vi "Analysis Configuration Dialog.vi"(11 "Data In":T1={"UI References"={"Exit Ref"=refnum, "Save Ref"=refnum, "Open Ref"=refnum, "Export Ref"=refnum, "Acquire Ref"=refnum, "Configure Ref"=refnum, "Graph Ref"=refnum, "Clear Ref"=refnum, "Analyze Ref"=refnum, "Status Ref"=refnum, "Snapshot Ref"=refnum}, "User Specified"={"Hardware Configuration"={"Signal Channel"="PXI1Slot7/ao0", "Response Channel"="PXI1Slot7/ai0", "Trigger Channel"="/PXI1Slot7/PFI0", "Number of Acquisitions"=1.0}, "Analysis Configuration"={"Statistics"=TRUE}, "Signal Type"=enum."From Excel", "New Data Behavior"=enum."Replace", "Signal Configuration"={"Chirp Amplitude"=0.0, "I/O Limit"=0.0, "Sample Rate"=0.0, "Chirp Duration (s)"=0.0, "Upper Frequency"=0.0, "Lower Frequency"=0.0, "Windowing"=enum."None"}, "Waveform File"="", "Save Location"=""}}) -> (3 "Data Out":T1={"UI References"={"Exit Ref"=refnum, "Save Ref"=refnum, "Open Ref"=refnum, "Export Ref"=refnum, "Acquire Ref"=refnum, "Configure Ref"=refnum, "Graph Ref"=refnum, "Clear Ref"=refnum, "Analyze Ref"=refnum, "Status Ref"=refnum, "Snapshot Ref"=refnum}, "User Specified"={"Hardware Configuration"={"Signal Channel"="PXI1Slot7/ao0", "Response Channel"="PXI1Slot7/ai0", "Trigger Channel"="/PXI1Slot7/PFI0", "Number of Acquisitions"=1.0}, "Analysis Configuration"={"Statistics"=TRUE}, "Signal Type"=enum."From Excel", "New Data Behavior"=enum."Replace", "Signal Configuration"={"Chirp Amplitude"=0.0, "I/O Limit"=0.0, "Sample Rate"=0.0, "Chirp Duration (s)"=0.0, "Upper Frequency"=0.0, "Lower Frequency"=0.0, "Windowing"=enum."None"}, "Waveform File"="", "Save Location"=""}})   [LabVIEW 2017]
doc: "Displays the analysis configuration dialog if the user has the \"Prompt?\" preference set."
uses:
  controls/Data.ctl
  controls/UI References.ctl
  controls/HW Configuration.ctl
  controls/Analysis Configuration.ctl
  controls/New Data Behavior.ctl
  controls/Signal Configuration.ctl
panel:
  # "(Scroll up to see large state data in/out clusters)"
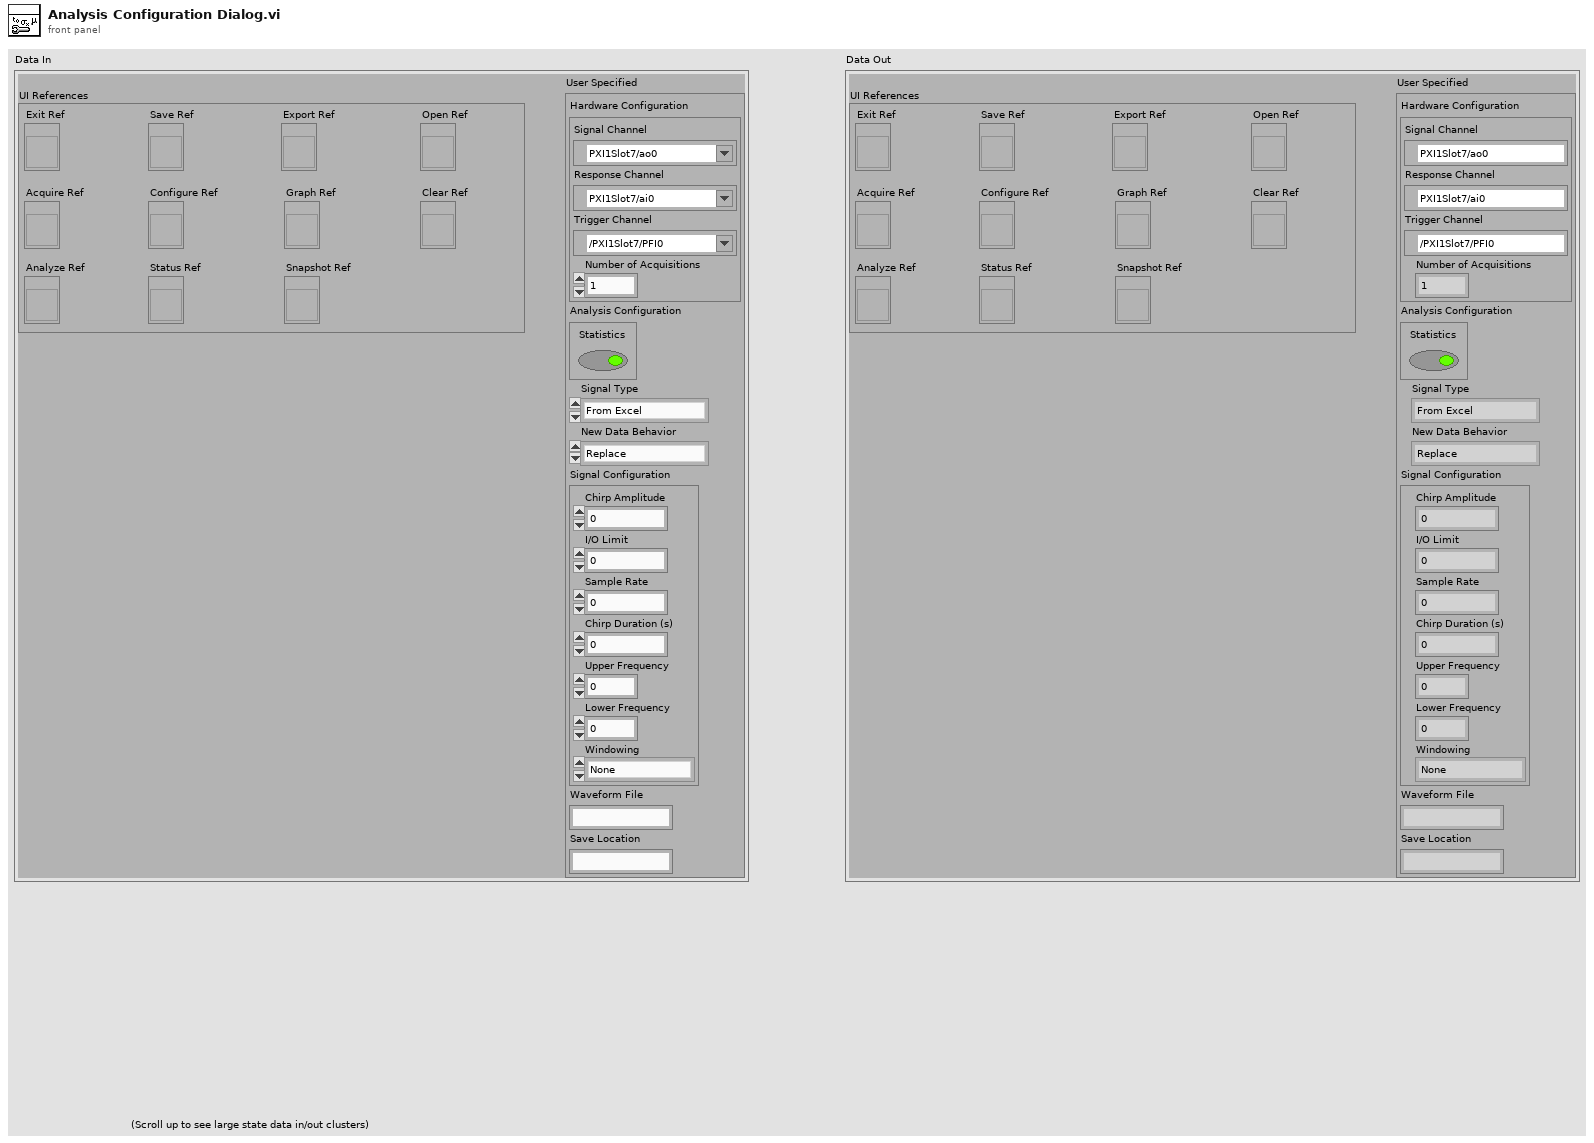
[diagram p1: front panel]
types:
  T1 = typedef "Data.ctl" = cluster{"UI References":T2, "User Specified":cluster{"Hardware Configuration":T3, "Analysis Configuration":T4, "Signal Type":enum16{"From Excel", "Single Chirp"}, "New Data Behavior":T5, "Signal Configuration":T6, "Waveform File":string, "Save Location":string}}
  T2 = typedef "UI References.ctl" = cluster{"Exit Ref":refnum<vi>, "Save Ref":refnum<vi>, "Open Ref":refnum<vi>, "Export Ref":refnum<vi>, "Acquire Ref":refnum<vi>, "Configure Ref":refnum<vi>, "Graph Ref":refnum<vi>, "Clear Ref":refnum<vi>, "Analyze Ref":refnum<vi>, "Status Ref":refnum<vi>, "Snapshot Ref":refnum<vi>}
  T3 = typedef "HW Configuration.ctl" = cluster{"Signal Channel":tag, "Response Channel":tag, "Trigger Channel":tag, "Number of Acquisitions":dbl}
  T4 = typedef "Analysis Configuration.ctl" = cluster{"Statistics":bool}
  T5 = typedef "New Data Behavior.ctl" = enum16{"Replace", "Overlay", "Append"}
  T6 = typedef "Signal Configuration.ctl" = cluster{"Chirp Amplitude":dbl, "I/O Limit":dbl, "Sample Rate":dbl, "Chirp Duration (s)":dbl, "Upper Frequency":dbl, "Lower Frequency":dbl, "Windowing":enum16{"None", "Exponential", "Flat top", "Hamming", "Hanning", "Kaiser-Bessel", "Rectangular"}}
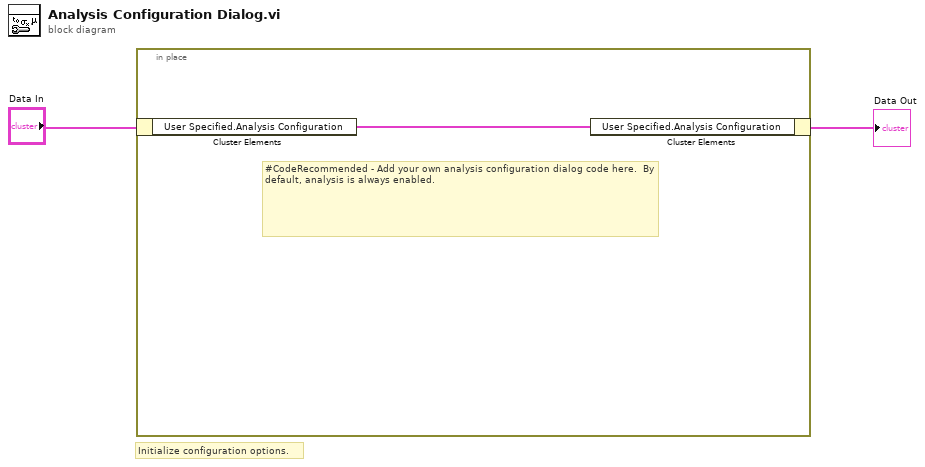
[diagram p0: block diagram]
diagram:
  # "Initialize configuration options."
  n1 = in-place {
    # "#CodeRecommended - Add your own analysis configuration dialog code here.  By default, analysis is always enabled."
    n2 = in-place-cluster #1("Data In") -> ("User Specified.Analysis Configuration"=w3:T4)
    n3 = in-place-cluster #1("User Specified.Analysis Configuration"=w3) -> (→"Data Out":T1)
  }
